vi "Min Pixels (SubVI).vi"(10 "Pixel Bundle 2":T1, 11 "Pixel Bundle 1":T1) -> (3 "Min Pixels":T1)   [LabVIEW 2015]
uses:
  Controls (FPGA)/Pixel Bundle (x16).ctl
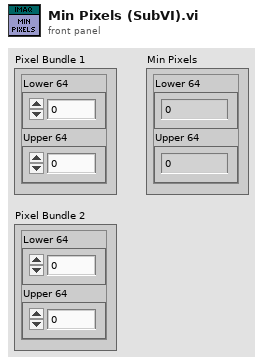
[diagram p1: front panel]
types:
  T1 = typedef "Pixel Bundle (x16).ctl" = cluster{"Lower 64":u64, "Upper 64":u64}
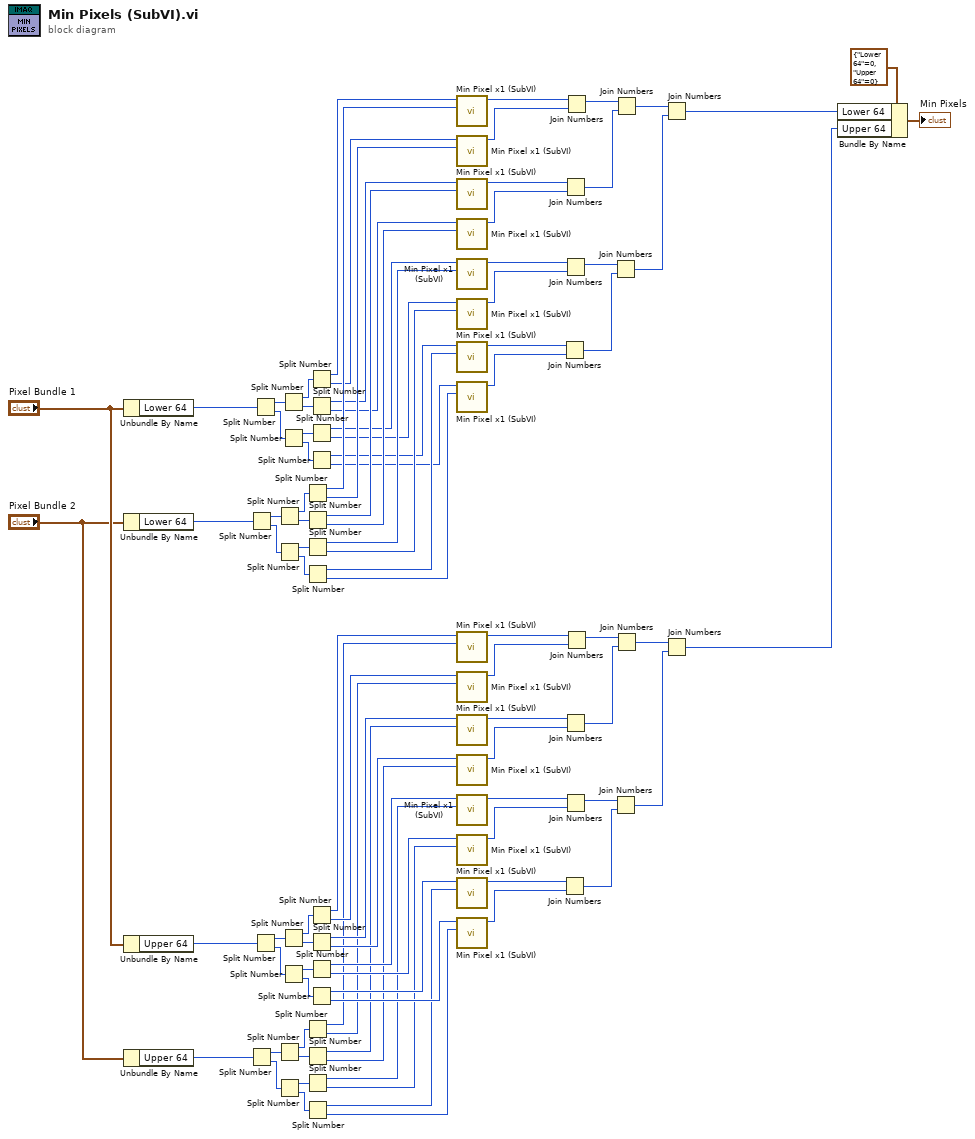
[diagram p0: block diagram]
diagram:
  n1 = Unbundle By Name("Pixel Bundle 1") -> ("Lower 64"=w94:u64)
  n2 = Unbundle By Name("Pixel Bundle 2") -> ("Lower 64"=w81:u64)
  n3 = Unbundle By Name("Pixel Bundle 1") -> ("Upper 64"=w6:u64)
  n4 = Unbundle By Name("Pixel Bundle 2") -> ("Upper 64"=w19:u64)
  n5 = Split Number(x=w81) -> (hi(x)=w83:u32, lo(x)=w82:u32)
  n6 = Split Number(x=w19) -> (hi(x)=w17:u32, lo(x)=w18:u32)
  n7 = Split Number(x=w94) -> (hi(x)=w92:u32, lo(x)=w93:u32)
  n8 = Split Number(x=w6) -> (hi(x)=w8:u32, lo(x)=w7:u32)
  n9 = Split Number(x=w83) -> (hi(x)=w85:u16, lo(x)=w84:u16)
  n10 = Split Number(x=w82) -> (hi(x)=w86:u16, lo(x)=w87:u16)
  n11 = Split Number(x=w17) -> (hi(x)=w15:u16, lo(x)=w16:u16)
  n12 = Split Number(x=w18) -> (hi(x)=w14:u16, lo(x)=w13:u16)
  n13 = Split Number(x=w92) -> (hi(x)=w90:u16, lo(x)=w91:u16)
  n14 = Split Number(x=w93) -> (hi(x)=w89:u16, lo(x)=w88:u16)
  n15 = Split Number(x=w8) -> (hi(x)=w10:u16, lo(x)=w9:u16)
  n16 = Split Number(x=w7) -> (hi(x)=w11:u16, lo(x)=w12:u16)
  n17 = Split Number(x=w85) -> (hi(x)=w79:u8, lo(x)=w77:u8)
  n18 = Split Number(x=w84) -> (hi(x)=w75:u8, lo(x)=w73:u8)
  n19 = Split Number(x=w86) -> (hi(x)=w71:u8, lo(x)=w69:u8)
  n20 = Split Number(x=w87) -> (hi(x)=w67:u8, lo(x)=w65:u8)
  n21 = Split Number(x=w15) -> (hi(x)=w21:u8, lo(x)=w23:u8)
  n22 = Split Number(x=w16) -> (hi(x)=w25:u8, lo(x)=w27:u8)
  n23 = Split Number(x=w14) -> (hi(x)=w29:u8, lo(x)=w31:u8)
  n24 = Split Number(x=w13) -> (hi(x)=w33:u8, lo(x)=w35:u8)
  n25 = Split Number(x=w90) -> (hi(x)=w80:u8, lo(x)=w78:u8)
  n26 = Split Number(x=w91) -> (hi(x)=w76:u8, lo(x)=w74:u8)
  n27 = Split Number(x=w89) -> (hi(x)=w72:u8, lo(x)=w70:u8)
  n28 = Split Number(x=w88) -> (hi(x)=w68:u8, lo(x)=w66:u8)
  n29 = Split Number(x=w10) -> (hi(x)=w20:u8, lo(x)=w22:u8)
  n30 = Split Number(x=w9) -> (hi(x)=w24:u8, lo(x)=w26:u8)
  n31 = Split Number(x=w11) -> (hi(x)=w28:u8, lo(x)=w30:u8)
  n32 = Split Number(x=w12) -> (hi(x)=w32:u8, lo(x)=w34:u8)
  n33 = call "Min Pixel x1 (SubVI).vi"("Pixel 2"=w79, "Pixel 1"=w80) -> ("Min Pixel"=w64:u8)  [unwired: 9 in]
  n34 = call "Min Pixel x1 (SubVI).vi"("Pixel 2"=w77, "Pixel 1"=w78) -> ("Min Pixel"=w63:u8)  [unwired: 9 in]
  n35 = call "Min Pixel x1 (SubVI).vi"("Pixel 2"=w75, "Pixel 1"=w76) -> ("Min Pixel"=w62:u8)  [unwired: 9 in]
  n36 = call "Min Pixel x1 (SubVI).vi"("Pixel 2"=w73, "Pixel 1"=w74) -> ("Min Pixel"=w61:u8)  [unwired: 9 in]
  n37 = call "Min Pixel x1 (SubVI).vi"("Pixel 2"=w71, "Pixel 1"=w72) -> ("Min Pixel"=w56:u8)  [unwired: 9 in]
  n38 = call "Min Pixel x1 (SubVI).vi"("Pixel 2"=w69, "Pixel 1"=w70) -> ("Min Pixel"=w55:u8)  [unwired: 9 in]
  n39 = call "Min Pixel x1 (SubVI).vi"("Pixel 2"=w67, "Pixel 1"=w68) -> ("Min Pixel"=w54:u8)  [unwired: 9 in]
  n40 = call "Min Pixel x1 (SubVI).vi"("Pixel 2"=w65, "Pixel 1"=w66) -> ("Min Pixel"=w53:u8)  [unwired: 9 in]
  n41 = call "Min Pixel x1 (SubVI).vi"("Pixel 2"=w21, "Pixel 1"=w20) -> ("Min Pixel"=w36:u8)  [unwired: 9 in]
  n42 = call "Min Pixel x1 (SubVI).vi"("Pixel 2"=w23, "Pixel 1"=w22) -> ("Min Pixel"=w37:u8)  [unwired: 9 in]
  n43 = call "Min Pixel x1 (SubVI).vi"("Pixel 2"=w25, "Pixel 1"=w24) -> ("Min Pixel"=w38:u8)  [unwired: 9 in]
  n44 = call "Min Pixel x1 (SubVI).vi"("Pixel 2"=w27, "Pixel 1"=w26) -> ("Min Pixel"=w39:u8)  [unwired: 9 in]
  n45 = call "Min Pixel x1 (SubVI).vi"("Pixel 2"=w29, "Pixel 1"=w28) -> ("Min Pixel"=w44:u8)  [unwired: 9 in]
  n46 = call "Min Pixel x1 (SubVI).vi"("Pixel 2"=w31, "Pixel 1"=w30) -> ("Min Pixel"=w45:u8)  [unwired: 9 in]
  n47 = call "Min Pixel x1 (SubVI).vi"("Pixel 2"=w33, "Pixel 1"=w32) -> ("Min Pixel"=w46:u8)  [unwired: 9 in]
  n48 = call "Min Pixel x1 (SubVI).vi"("Pixel 2"=w35, "Pixel 1"=w34) -> ("Min Pixel"=w47:u8)  [unwired: 9 in]
  n49 = Join Numbers(hi=w54, lo=w53) -> ((hi.lo)=w58:u16)
  n50 = Join Numbers(hi=w46, lo=w47) -> ((hi.lo)=w42:u16)
  n51 = Join Numbers(hi=w62, lo=w61) -> ((hi.lo)=w59:u16)
  n52 = Join Numbers(hi=w56, lo=w55) -> ((hi.lo)=w57:u16)
  n53 = Join Numbers(hi=w38, lo=w39) -> ((hi.lo)=w41:u16)
  n54 = Join Numbers(hi=w44, lo=w45) -> ((hi.lo)=w43:u16)
  n55 = Join Numbers(hi=w64, lo=w63) -> ((hi.lo)=w60:u16)
  n56 = Join Numbers(hi=w36, lo=w37) -> ((hi.lo)=w40:u16)
  n57 = Join Numbers(hi=w57, lo=w58) -> ((hi.lo)=w51:u32)
  n58 = Join Numbers(hi=w43, lo=w42) -> ((hi.lo)=w49:u32)
  n59 = Join Numbers(hi=w60, lo=w59) -> ((hi.lo)=w52:u32)
  n60 = Join Numbers(hi=w40, lo=w41) -> ((hi.lo)=w48:u32)
  n61 = Join Numbers(hi=w52, lo=w51) -> ((hi.lo)=w50:u64)
  n62 = Join Numbers(hi=w48, lo=w49) -> ((hi.lo)=w5:u64)
  n63 = Bundle By Name(cluster=T1 {"Lower 64"=0, "Upper 64"=0} ("Pixel Bundle (x16)"), "Lower 64"=w50, "Upper 64"=w5) -> (→"Min Pixels":T1)
